vi "ExampleEvent.vi"() -> ()   [LabVIEW 2020]
panel:
  out "error out":errorcluster
  in  "error in (no error)":errorcluster
  in  "stop":bool
  in  "Button 3":bool
  in  "Button 2":bool
  in  "Button 1":bool
  # "NOTE :\n\n<Mechanical Action>\n\nButton for Event Structure  - Latch\nButton for While Loop - Switch"
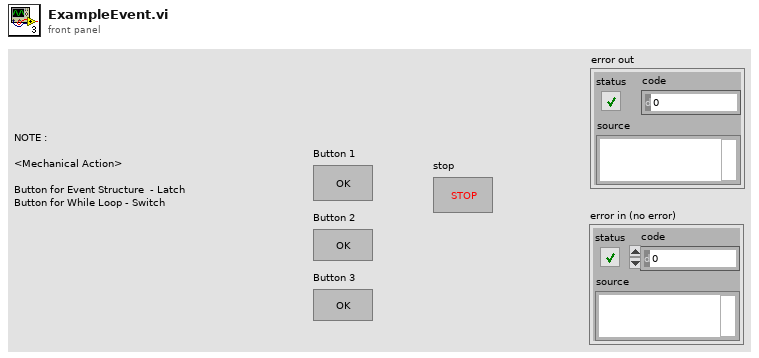
[diagram p1: front panel]
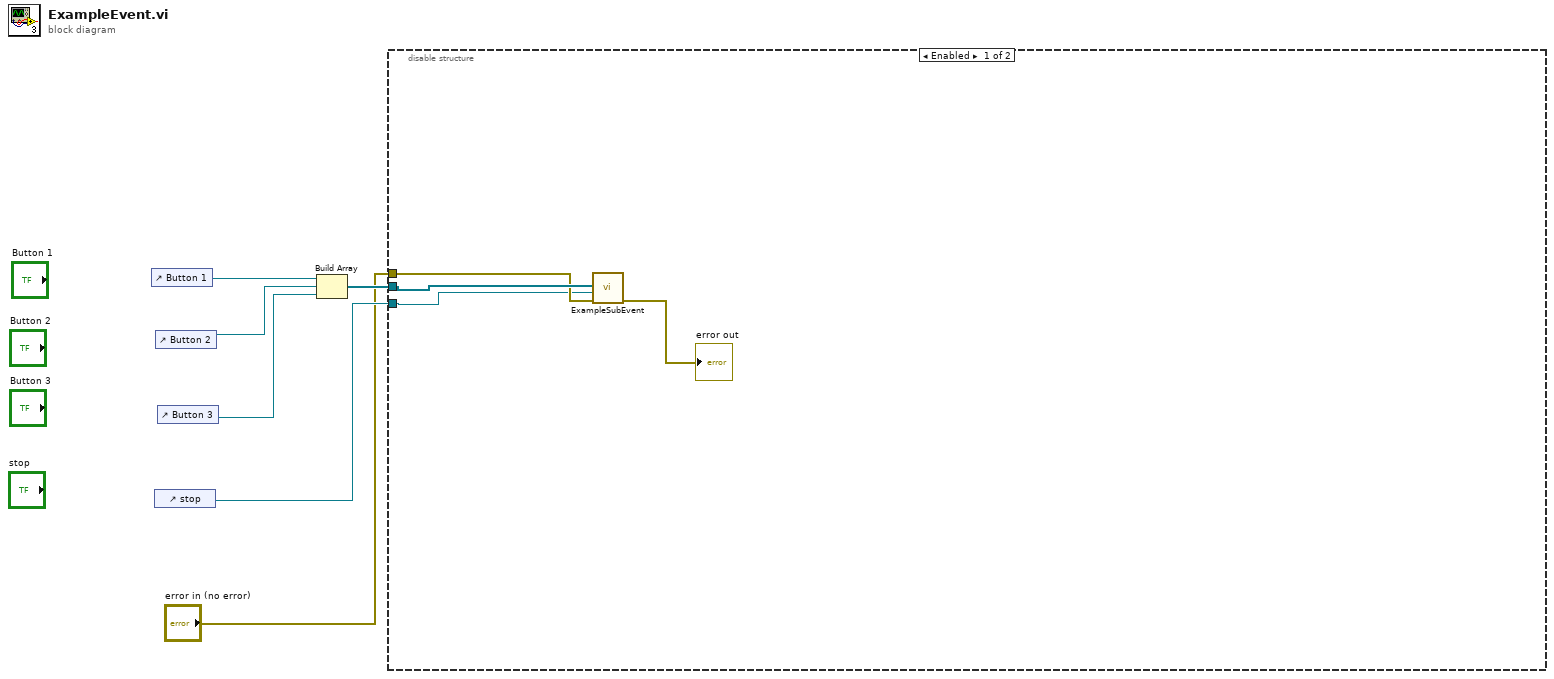
[diagram p0: block diagram]
diagram:
  n1 = control-ref of="Button 1"() -> (w6:refnum<vi>)
  n2 = control-ref of="stop"() -> (w2:refnum<vi>)
  n3 = control-ref of="Button 2"() -> (w5:refnum<vi>)
  n4 = control-ref of="Button 3"() -> (w4:refnum<vi>)
  n5 = Build Array(w6, w5, w4) -> (w3:refnum<vi>[])
  n6 = disable-structure shown="Enabled" {
    disable-tunnel: w3 -> [w10 _]
    disable-tunnel: w2 -> [w7 _]
    disable-tunnel: "error in (no error)" -> [w9 _]
    frame Enabled {
      n7 = call "ExampleSubEvent.vi"("error in (no error)"=w9, "Stop Button event source"=w7, "Button Array event source"=w10) -> ("error out"=→"error out":errorcluster)  [unwired: 7 in]
    }
    frame Disabled {
    }
  }
